vi "Status Message_Display.vi"(6 "Add Timestamp (?)":bool=TRUE, 7 "QRD":T1, 8 "error in":errorcluster, 11 "Status Message":string) -> (0 "error out":errorcluster, 5 "QRD Out":T1)   [LabVIEW 2025]
uses:
  Controls/Queues-Refs-Data.ctl
  Builds/Queue Wrappers.lvlibp/Q Packet.ctl
  <vilib>/Utility/error.llb/whitespace.ctl
  <vilib>/Utility/error.llb/Trim Whitespace One-Sided.vi
  Builds/Queue Wrappers.lvlibp
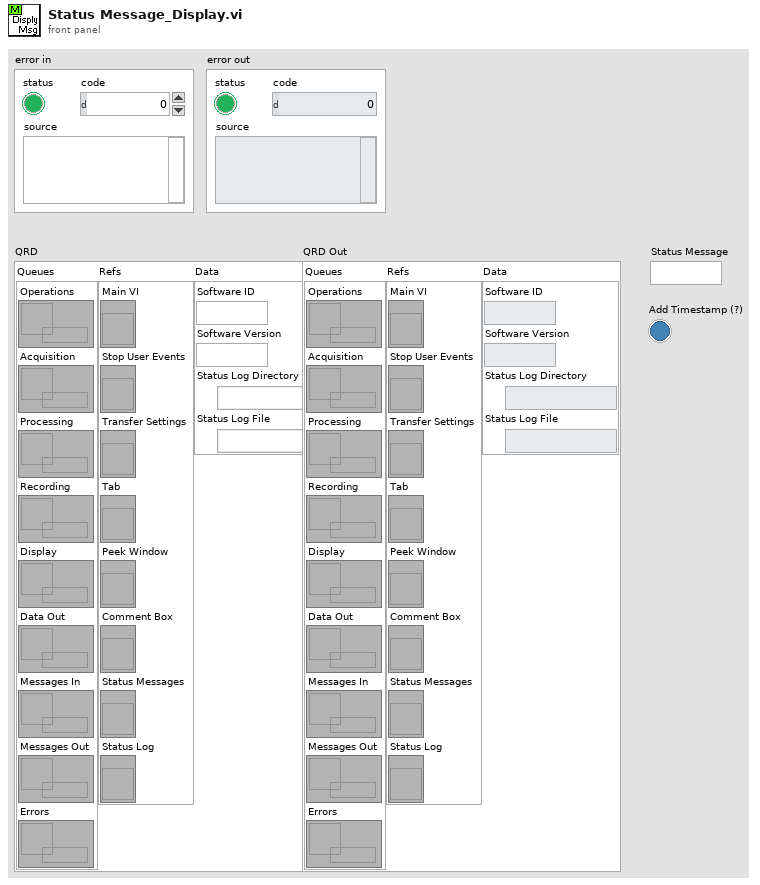
[diagram p1: front panel]
types:
  T1 = typedef "Queues-Refs-Data.ctl" = cluster{"Queues":cluster{"Operations":refnum<queue>, "Acquisition":refnum<queue>, "Processing":refnum<queue>, "Recording":refnum<queue>, "Display":refnum<queue>, "Data Out":refnum<queue>, "Messages In":refnum<queue>, "Messages Out":refnum<queue>, "Errors":refnum<queue>}, "Refs":cluster{"Main VI":refnum<vi>, "Stop User Events":refnum<vi>, "Transfer Settings":refnum<vi>, "Tab":refnum<vi>, "Peek Window":refnum<vi>, "Comment Box":refnum<vi>, "Status Messages":refnum<vi>, "Status Log":refnum<vi>}, "Data":cluster{"Software ID":string, "Software Version":string, "Status Log Directory":path, "Status Log File":path}}
  T2 = typedef "whitespace.ctl" = u16
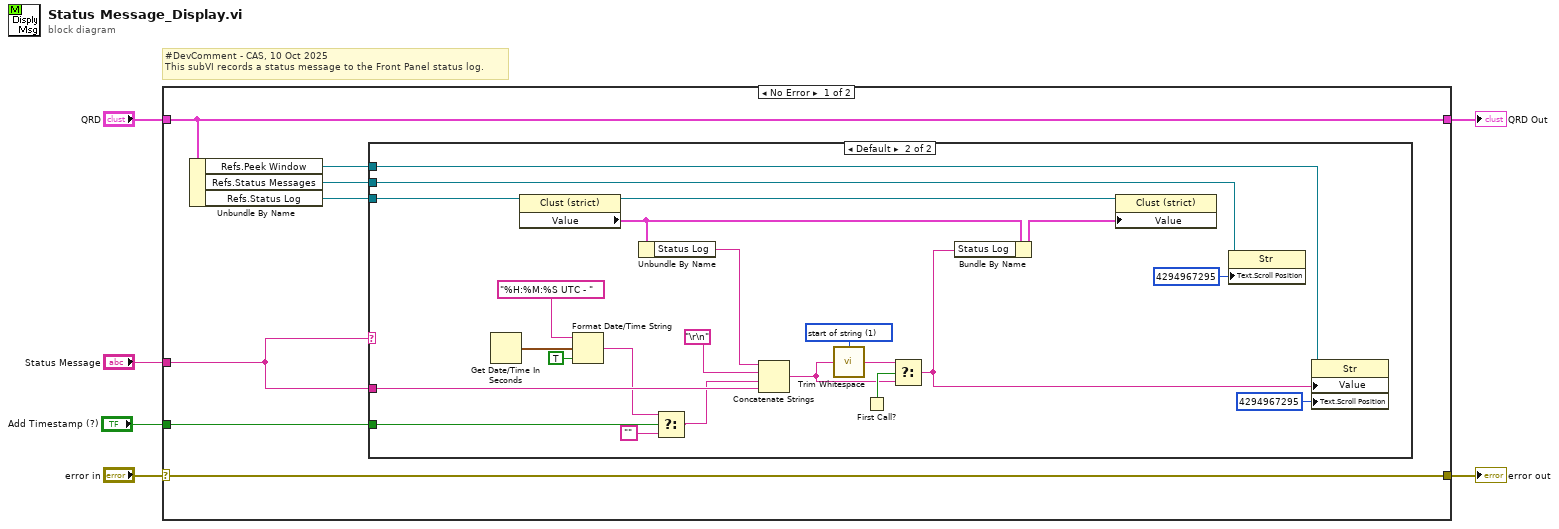
[diagram p0: block diagram]
diagram:
  # "#DevComment - CAS, 10 Oct 2025\nThis subVI records a status message to the Front Panel status log."
  n1 = case shown="No Error" "error in" {
    selector: "error in" -> [w13 w37]
    tunnel: "QRD" -> [w12 w38]
    tunnel: [w12 w38] -> w5
    tunnel: [w13 w37] -> w4
    tunnel: "Status Message" -> [w10 _]
    tunnel: "Add Timestamp (?)" -> [w9 _]
    frame No Error {
      n2 = Unbundle By Name(w12) -> ("Refs.Peek Window"=w7:refnum<vi>, "Refs.Status Messages"=w8:refnum<vi>, "Refs.Status Log"=w11:refnum<vi>)
      n3 = case shown="Default" w10 {
        tunnel: w11 -> [_ w33]
        tunnel: w10 -> [_ w29]
        tunnel: w9 -> [_ w21]
        tunnel: w8 -> [_ w18]
        tunnel: w7 -> [_ w16]
        frame "" {
        }
        frame Default {
          w24 = T2 1 items=["both", "start of string", "end of string"] ("location (both)")
          n4 = Get Date/Time In Seconds() -> (seconds since 1Jan1904=w36:timestamp)
          n5 = property class="Clust (strict)"(reference=w33) -> (reference out=w32:refnum<vi>, "Value"=w30:cluster{"Status Log":string, "Path":path})  [unwired: 1 in, 1 out]
          n6 = Format Date/Time String(time format string (%c)="%H:%M:%S UTC - ", seconds (now)=w36, UTC format=TRUE) -> (date/time string=w22:string)
          n7 = Unbundle By Name(w30) -> ("Status Log"=w28:string)
          n8 = Select(t=w22, s=w21, f="") -> (s? t:f=w19:string)
          n9 = Concatenate Strings(w28, "\r\n", w19, w29) -> (w23:string)
          n10 = call <vilib>:"Trim Whitespace.vi"("string"=w23, "location (both)"=w24) -> ("trimmed string"=w25:string)
          n11 = First Call?() -> (First Call?: T/F=w26:bool)
          n12 = Select(t=w25, s=w26, f=w23) -> (s? t:f=w15:string)
          n13 = Bundle By Name(cluster=w30, "Status Log"=w15) -> (w31:cluster{"Status Log":string, "Path":path})
          n14 = property class="Clust (strict)"(reference=w32, "Value"=w31) -> ()  [unwired: 1 in, 2 out]
          n15 = property class="Str"(reference=w18, "Text.Scroll Position"=u32 4294967295) -> ()  [unwired: 1 in, 2 out]
          n16 = property class="Str"(reference=w16, "Value"=w15, "Text.Scroll Position"=u32 4294967295) -> ()  [unwired: 1 in, 2 out]
        }
      }
    }
    frame Error {
    }
  }
  "error out" <- w4
  "QRD Out" <- w5
